vi "ADCP_Verify_Checksum_Raw_Packet.vi"(8 "error in (no error)":errorcluster, 10 "Raw Packet":u8[](array[numeric]), 11 "ADCP in":refnum<class "ADCP.lvclass">) -> (0 "error out":errorcluster, 2 "Checksum Valid ?":bool, 3 "ADCP out":refnum<class "ADCP.lvclass">)   [LabVIEW 2017, in "ADCP.lvclass"]
uses:
  ADCP.lvclass
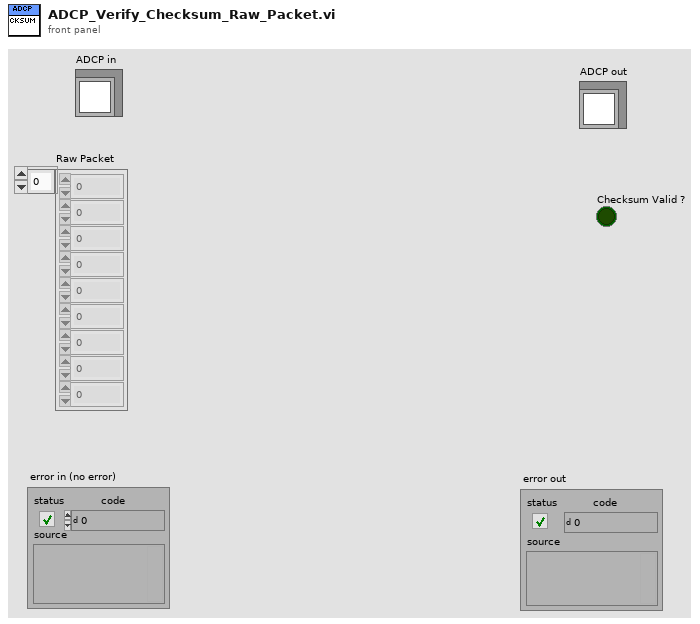
[diagram p1: front panel]
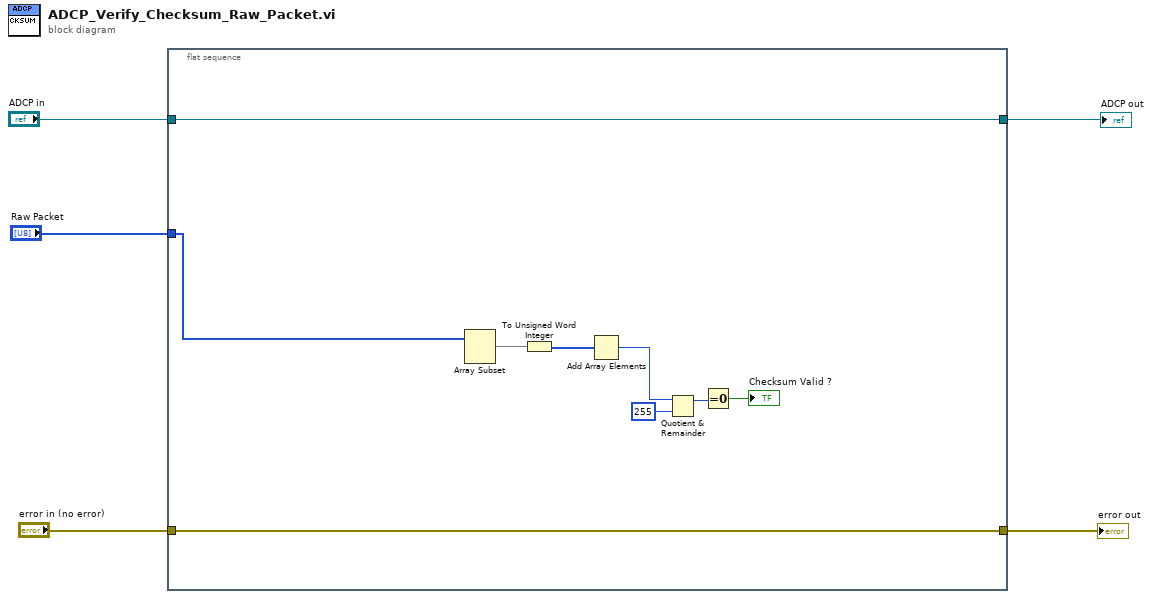
[diagram p0: block diagram]
diagram:
  n1 = flat-sequence {
    tunnel: "ADCP in" -> [w8]
    tunnel: "Raw Packet" -> [w7]
    tunnel: "error in (no error)" -> [w6]
    tunnel: [w8] -> w2
    tunnel: [w6] -> w1
    frame #0 {
      n2 = Array Subset(array=w7) -> (w14:u8[])  [unwired: 2 in]
      n3 = To Unsigned Word Integer(number=w14) -> (unsigned 16bit integer=w13:u16[])
      n4 = Add Array Elements(numeric array=w13) -> (sum=w12:u16)
      n5 = Quotient & Remainder(x=w12, y=u16 255) -> (x-y*floor(x/y)=w10:u16)  [unwired: 1 out]
      n6 = Equal To 0?(x=w10) -> (x = 0?=→"Checksum Valid ?":bool)
    }
  }
  "ADCP out" <- w2
  "error out" <- w1
